vi "Comments.Add Sweep Description.vi"(8 "error in (no error)":errorcluster, 11 "Control Experiment in":refnum<class "Control Experiment.lvclass">) -> (0 "error out":errorcluster, 2 "Sweep Description":string, 3 "Control Experiment out":refnum<class "Control Experiment.lvclass">)   [LabVIEW 2019, in "Control Experiment.lvclass"]
uses:
  Control Experiment.lvclass
  Control Experiment.lvclass/Control Experiment.ctl
  <userlib>/LevyLab/PLYM/YAML.lvclass
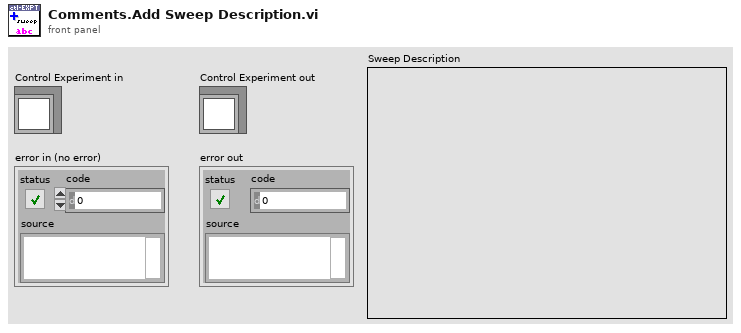
[diagram p1: front panel]
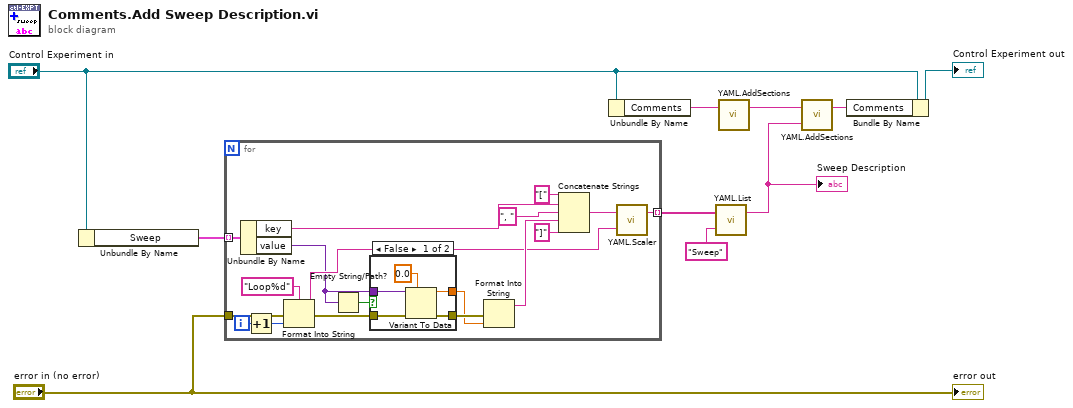
[diagram p0: block diagram]
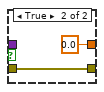
[diagram p2: hidden frame]
diagram:
  n1 = Unbundle By Name("Control Experiment in") -> ("Sweep"=w7:cluster{"key":string, "value":variant}[])
  n2 = for {
    tunnel: w7 -> [w28] mode=indexing
    tunnel: "error in (no error)" -> [w24]
    tunnel: [w22] -> w5 mode=indexing
    i -> [w27]
    n3 = Unbundle By Name(w28) -> ("key"=w20:string, "value"=w13:variant)
    n4 = Increment(x=w27) -> (x+1=w11:i32)
    n5 = Format Into String(format string="Loop%d" ("string"), error in=w24, w11) -> (resulting string=w14:string, error out=w23:errorcluster)  [unwired: 1 in]
    n6 = Empty String/Path?(string/path=w13) -> (empty?=w12:bool)
    n7 = case shown="False" w12 {
      tunnel: [w32 w35] -> w25
      tunnel: w23 -> [w31 w35]
      tunnel: w13 -> [w30 _]
      tunnel: [w29 0.0] -> w15
      frame False {
        n8 = Variant To Data(error in=w31, type=0.0, Variant=w30) -> (data=w29:dbl, error out=w32:errorcluster)
      }
      frame True {
      }
    }
    n9 = Format Into String(error in=w25, w15) -> (resulting string=w16:string)  [unwired: 2 in, 1 out]
    n10 = Concatenate Strings("[" ("string"), w20, ", " ("string"), w16, "]" ("string")) -> (w21:string)
    n11 = call <userlib>:"YAML.Scaler.vi"("Key"=w14, "Scaler"=w21) -> ("Output"=w22:string)  [unwired: 1 in]
  }
  n12 = Unbundle By Name("Control Experiment in") -> ("Comments"=w2:string)
  n13 = call <userlib>:"YAML.List.vi"("Key"="Sweep" ("string"), "lines"=w5) -> ("Output"=w3:string)  [unwired: 1 in]
  "Sweep Description" <- w3
  n14 = call <userlib>:"YAML.AddSections.vi"("Section 1"=w2) -> ("Output"=w1:string)  [unwired: 2 in]
  n15 = call <userlib>:"YAML.AddSections.vi"("Section 2"=w3, "Section 1"=w1) -> ("Output"=w10:string)  [unwired: 1 in]
  n16 = Bundle By Name(cluster="Control Experiment in", "Comments"=w10) -> (→"Control Experiment out":refnum<class "Control Experiment.lvclass">)
  "error out" <- "error in (no error)"
